vi "Open_Task.vi"(8 "error in (no error)":errorcluster caption="entrée d'erreur (pas d'erreur)", 11 "Class Log_File (Default) en entrée":refnum<class "Class Log_File (Default).lvclass">) -> (0 "error out":errorcluster caption="sortie d'erreur", 3 "Class Log_File (Default) en sortie":refnum<class "Class Log_File (Default).lvclass">)   [LabVIEW 2020, in "Library Instrument & Equipement.lvlib" / "Library Log_File.lvlib" / "Class Log_File (Default).lvclass"]
uses:
  Class Log_File (Default).lvclass
  Class Log_File (Default).lvclass/Class Log_File (Default).ctl
  Read CSV File/CSV_File (Default)/Class CSV_File.lvclass
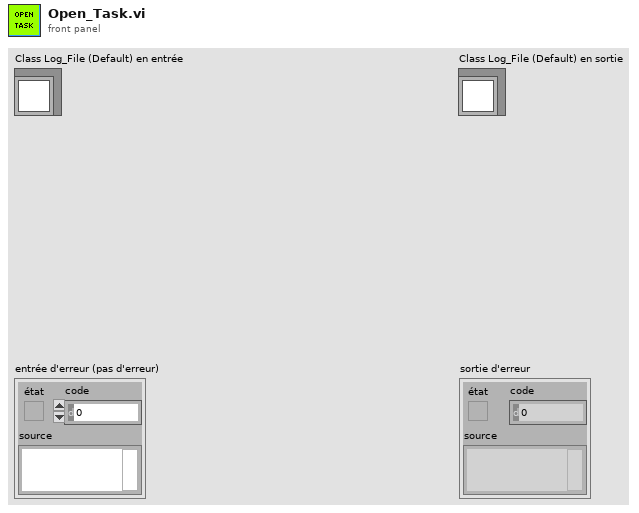
[diagram p1: front panel]
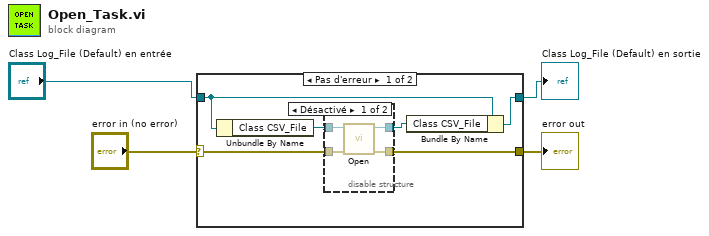
[diagram p0: block diagram]
diagram:
  n1 = case shown="Pas d'erreur" "error in (no error)" {
    selector: "error in (no error)" -> [w9 w18]
    tunnel: [w8 w18] -> w3
    tunnel: [w5 w17] -> w1
    tunnel: "Class Log_File (Default) en entrée" -> [w6 w17]
    frame No Error {
      n2 = Unbundle By Name(w6) -> ("Class CSV_File"=w10:refnum<class "Class CSV_File.lvclass">)
      n3 = disable-structure shown="Désactivé" {
        disable-tunnel: w10 -> [w14 w15]
        disable-tunnel: w9 -> [w13 w16]
        disable-tunnel: [w12 w16] -> w8
        disable-tunnel: [w11 w15] -> w7
        frame Disabled {
          n4 = call-dynamic "Open.vi"("error in (no error)"=w13, "Class CSV_File (Default) en entrée"=w14) -> ("error out"=w12:errorcluster, "Class CSV_File (Default) en sortie"=w11:refnum<class "Class CSV_File.lvclass">)  [unwired: 8 in]
        }
        frame Enabled {
        }
      }
      n5 = Bundle By Name(cluster=w6, "Class CSV_File"=w7) -> (w5:refnum<class "Class Log_File (Default).lvclass">)
    }
    frame Error {
    }
  }
  "error out" <- w3
  "Class Log_File (Default) en sortie" <- w1
